vi "Example_Game.vi"() -> ()   [LabVIEW 2015]
uses:
  TronviewGame/Game/GameResult.ctl
  TronviewGame/Board/BoardSize.ctl
  TronviewGame/Board/Board.lvclass
  TronviewGame/Player/Player.lvclass
  TronviewGame/TronviewGame.lvlib
  TronviewGame/GameRecorder/GameRecorder.lvclass
  TronviewGame/Game/Game.lvclass
panel:
  out "GameString":string
  out "GameResult":T1
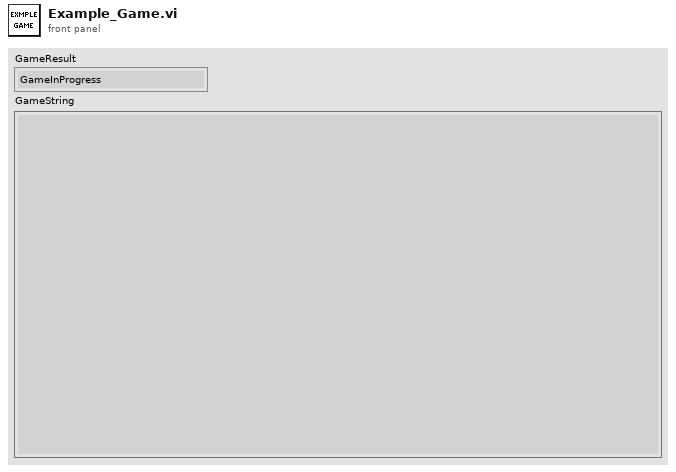
[diagram p1: front panel]
types:
  T1 = typedef "TronviewGame.lvlib/Game.lvclass/GameResult.ctl" = enum16{"GameInProgress", "Draw", "Player1Won", "Player2Won"}
  T2 = typedef "TronviewGame.lvlib/Board.lvclass/BoardSize.ctl" = cluster{"Columns":u16, "Rows":u16}
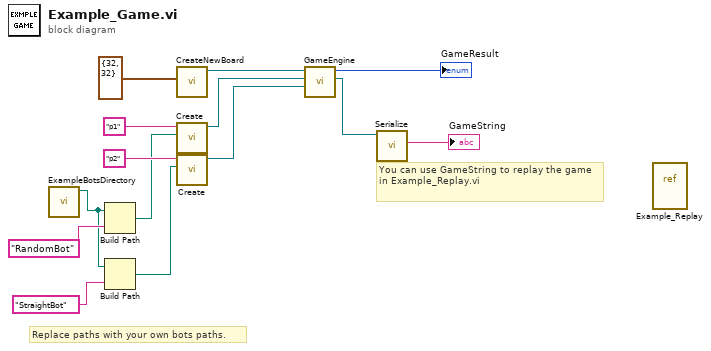
[diagram p0: block diagram]
diagram:
  # "Replace paths with your own bots paths."
  # "You can use GameString to replay the game in Example_Replay.vi"
  n1 = call "ExampleBotsDirectory.vi"() -> ("stripped path"=w10:path)  [unwired: 11 in]
  n2 = Build Path(base path=w10, name or relative path="RandomBot") -> (appended path=w1:path)
  n3 = Build Path(base path=w10, name or relative path="StraightBot") -> (appended path=w8:path)
  n4 = call "CreateNewBoard.vi"("Size"=T2 {"Columns"=32, "Rows"=32}) -> ("Board out"=w7:refnum<class "Board.lvclass">)  [unwired: 9 in, 1 out]
  n5 = call "Create.vi"("PlayerFolder"=w1, "PlayerName"="p1") -> ("Player out"=w6:refnum<class "Player.lvclass">)  [unwired: 8 in, 1 out]
  n6 = call "Create.vi"("PlayerFolder"=w8, "PlayerName"="p2") -> ("Player out"=w5:refnum<class "Player.lvclass">)  [unwired: 8 in, 1 out]
  n7 = call "GameEngine.vi"("Player2"=w5, "Player1"=w6, "Board"=w7) -> ("GameRecord"=w4:refnum<class "GameRecorder.lvclass">, "GameResult"=→"GameResult":T1)  [unwired: 6 in, 1 out]
  n8 = call "Serialize.vi"("GameRecorder in"=w4) -> ("String"=→"GameString":string)  [unwired: 8 in, 2 out]
  n9 = vi-ref "Example_Replay.vi"() -> ()  [unwired: 1 out]
